vi "Write Secrets.vi"(8 "error in (no error)":errorcluster, 10 "Secrets":string, 11 "Test Dialog Return Msg in":refnum<class "Test Dialog Return Msg.lvclass">) -> (0 "error out":errorcluster, 3 "Test Dialog Return Msg out":refnum<class "Test Dialog Return Msg.lvclass">)   [LabVIEW 2018, in "TopLevelApplication.lvlib" / "Test Dialog Return Msg.lvclass"]
doc: "<License>\nCopyright © 2017 Composed Systems, LLC | All rights reserved\nwww.composed.io\n\nAuthor: Ethan Stern <ethan.stern@composed.io>\n\nThis software is provided \"AS IS\" WITHOUT WARRANTIES, either express or implied, AND IS FOR EDUCATIONAL PURPOSES ONLY.\n</License>"
uses:
  Test Dialog Return Msg.lvclass
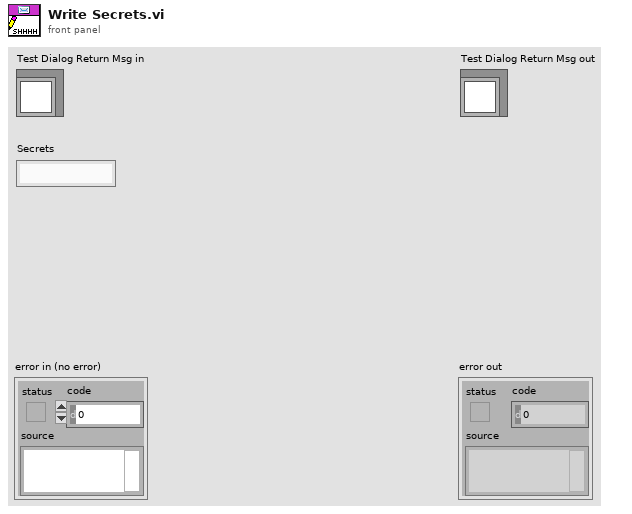
[diagram p1: front panel]
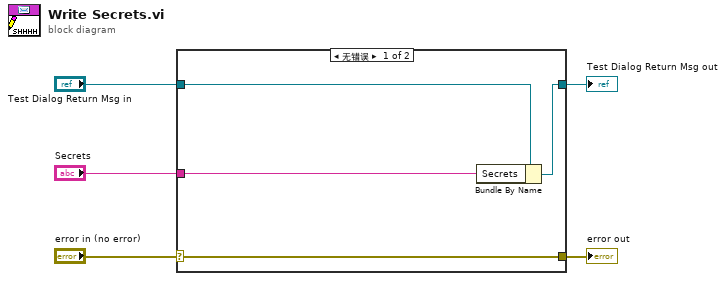
[diagram p0: block diagram]
diagram:
  n1 = case shown="无错误" "error in (no error)" {
    selector: "error in (no error)" -> [w9 w10]
    tunnel: [w9 w10] -> w4
    tunnel: [w7 w11] -> w2
    tunnel: "Test Dialog Return Msg in" -> [w8 w11]
    tunnel: "Secrets" -> [w6 _]
    frame No Error {
      n2 = Bundle By Name(cluster=w8, "Secrets"=w6) -> (w7:refnum<class "Test Dialog Return Msg.lvclass">)
    }
    frame Error {
    }
  }
  "error out" <- w4
  "Test Dialog Return Msg out" <- w2
